vi "Stop Core.vi"(10 "final error code":i32, 11 "Syringe in":refnum<class "Syringe Line.lvclass">) -> (3 "Syringe out":refnum<class "Syringe Line.lvclass">)   [LabVIEW 2015, in "cRIO-Carbondioxide.lvlib" / "CO2-Actor.lvlib" / "Syringe Line.lvclass"]
doc: "(<B>Filename</B>: Actor Framework.lvlib:Actor.lvclass:Stop Core.vi)\n\nDefines what the actor does before it stops. Use the <B>final error code</B> input to determine whether the actor shut down in response to an error.\n\nBy default, this method does nothing. A descendant class may override it to define behavior, such as shutting down any processes the actor initiated in its override of the Actor Core method."
uses:
  Syringe Line.lvclass
  Syringe Line.lvclass/Syringe Line.ctl
  CO2 Actor/CO2 Actor.lvclass
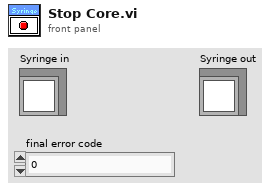
[diagram p1: front panel]
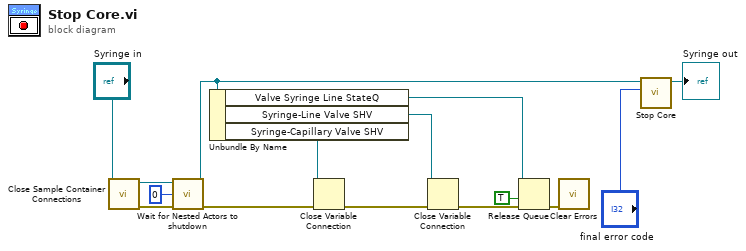
[diagram p0: block diagram]
diagram:
  n1 = call "Close Sample Container Connections.vi"("Syringe in"="Syringe in") -> ("error out"=w5:errorcluster, "Syringe out"=w2:refnum<class "Syringe Line.lvclass">)  [unwired: 9 in]
  n2 = call-dynamic "Wait for Nested Actors to shutdown.vi"("error in (no error)"=w5, "Timeout (-1)"=0, "Syringe Line in"=w2) -> ("error out"=w4:errorcluster, "Syringe Line out"=w3:refnum<class "Syringe Line.lvclass">)  [unwired: 7 in]
  n3 = Unbundle By Name(w3) -> ("Valve Syringe Line StateQ"=w9:refnum<queue>, "Syringe-Line Valve SHV"=w10:refnum<k21>, "Syringe-Capillary Valve SHV"=w12:refnum<k21>)
  n4 = Close Variable Connection(8:w4, 11:w12) -> (0:w11:errorcluster)
  n5 = Close Variable Connection(8:w11, 11:w10) -> (0:w8:errorcluster)
  n6 = Release Queue(queue=w9, force destroy? (F)=TRUE, error in (no error)=w8) -> (error out=w6:errorcluster)  [unwired: 2 out]
  n7 = call <vilib>:"Clear Errors.vi"("error in (no error)"=w6) -> ()  [unwired: 5 in, 2 out]
  n8 = call-parent "Stop Core.vi"("final error code"="final error code", "CO2 Actor in"=w3) -> ("CO2 Actor out"=→"Syringe out":refnum<class "Syringe Line.lvclass">)  [unwired: 9 in]
